vi "Extract Latest.vi"(8 "Error":errorcluster, 10 "Raw Data Waveform":T1, 11 "((Pointer))":refnum<class "_Pointer.lvclass">) -> (0 "Error Out":errorcluster, 2 "Waveform Out":T1, 3 "((Pointer)) Out":refnum<class "_Pointer.lvclass">)   [LabVIEW 2025, in "_Pointer.lvclass"]
uses:
  _Pointer.lvclass
  Universal Controls/Waveform_Data.ctl
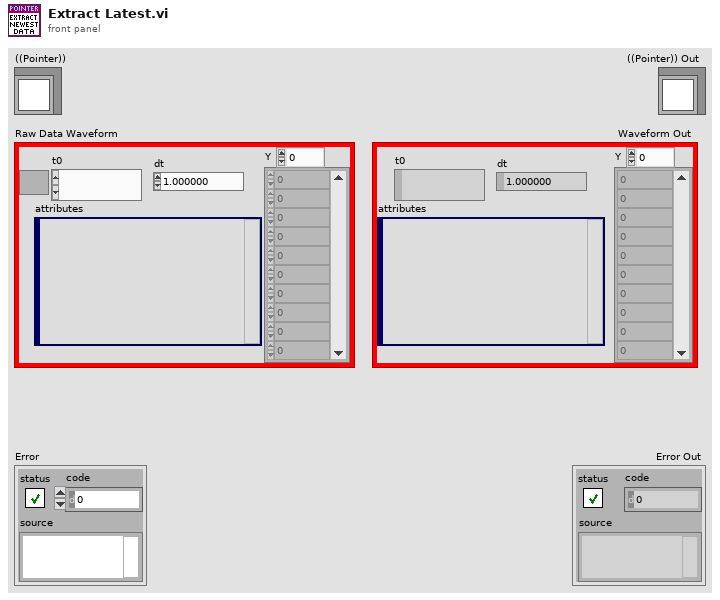
[diagram p1: front panel]
types:
  T1 = typedef "Waveform_Data.ctl" = waveform(dbl)
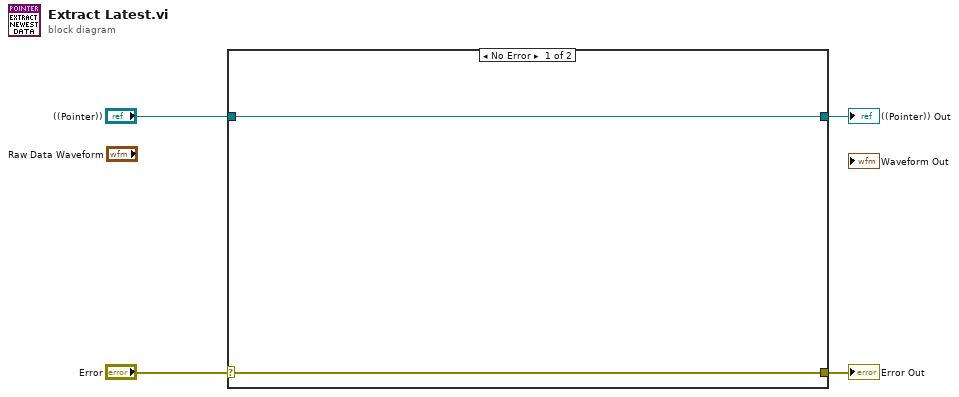
[diagram p0: block diagram]
diagram:
  n1 = case shown="No Error" "Error" {
    selector: "Error" -> [w5 w8]
    tunnel: [w5 w8] -> w3
    tunnel: [w6 w7] -> w1
    tunnel: "((Pointer))" -> [w6 w7]
    frame No Error {
    }
    frame Error {
    }
  }
  "Error Out" <- w3
  "((Pointer)) Out" <- w1
